vi "Is Expected Filename.vi"(1 "Filename":string) -> (0 "Matches the expected settings filename?":bool)   [LabVIEW 2022 SP3]
doc: "This VI returns True if and only if the input Filename (including file extension) matches the expected settings file filename."
uses:
  <vilib>/Utility/error.llb/Trim Whitespace One-Sided.vi
panel:
  # "Development\nControls or indicators that are useful for development or testing, but which are not outputs of the VI."
  # "Input\nInputs to the VI"
  # "Output\nOutputs of the VI"
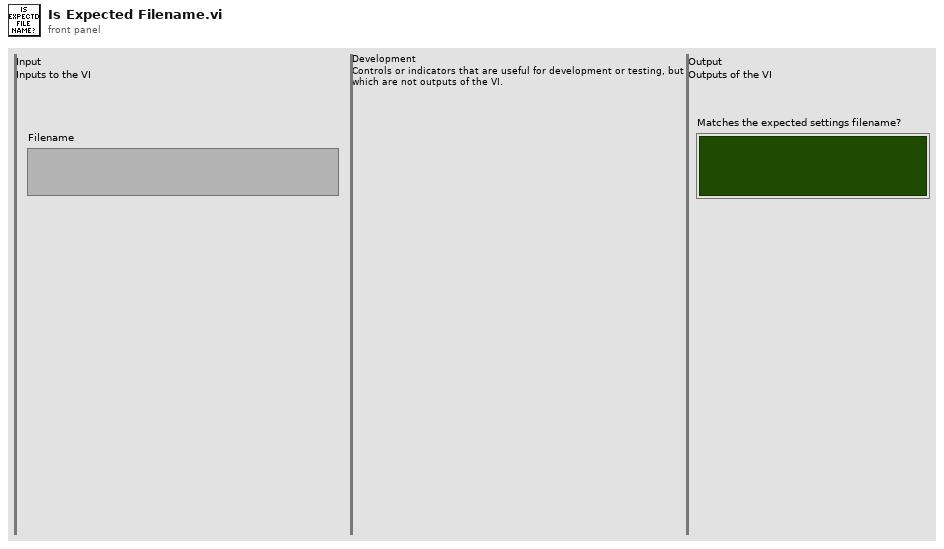
[diagram p1: front panel]
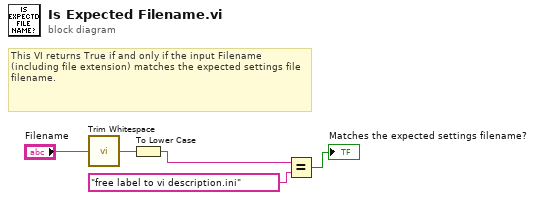
[diagram p0: block diagram]
diagram:
  # "This VI returns True if and only if the input Filename (including file extension) matches the expected settings file filename."
  n1 = call <vilib>:"Trim Whitespace.vi"("string"="Filename") -> ("trimmed string"=w5:string)  [unwired: 1 in]
  n2 = To Lower Case(string=w5) -> (all lower case string=w4:string)
  n3 = Equal?(x=w4, y="free label to vi description.ini") -> (x = y?=→"Matches the expected settings filename?":bool)
